vi "AttCtrlThruster.vi"(0 "ctclk":bool, 1 "Duty Cycle":dbl=1.0, 2 "Up":bool, 3 "Period":dbl=10.0, 4 "clkwis":bool, 5 "Float":bool, 6 "Angular Acceleration":u16(ring) items=["Fast", "Slow"], 7 "Left":bool, 8 "Right":bool, 9 "task in":refnum<k21>, 11 "error in":errorcluster, 13 "Down":bool) -> (10 "task out":refnum<k21>, 15 "error out":errorcluster)   [LabVIEW 2012]
panel:
  # "Attitude Control"
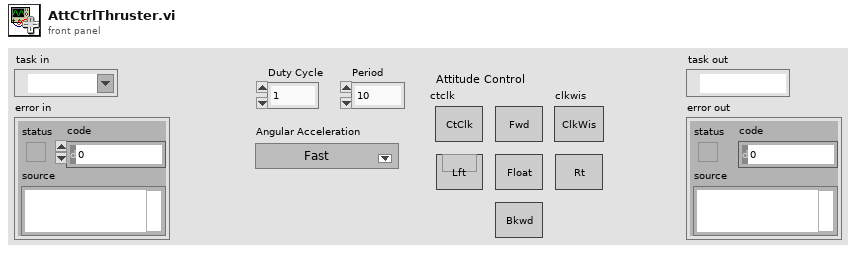
[diagram p1: front panel]
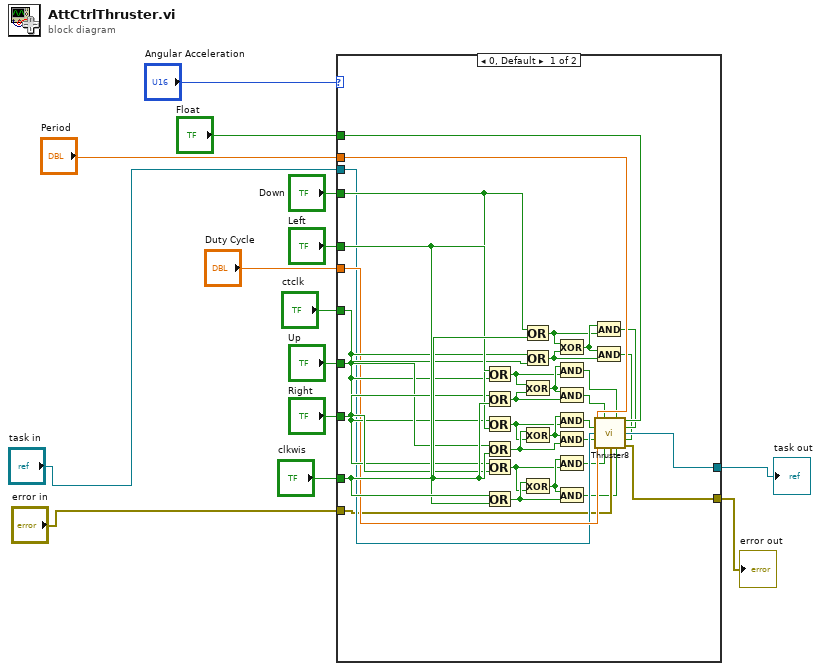
[diagram p0: block diagram]
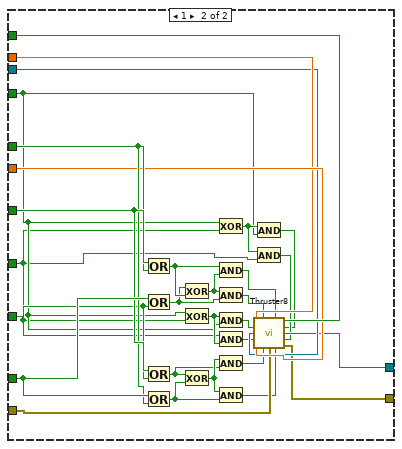
[diagram p2: hidden frame]
diagram:
  n1 = case shown="0, Default" "Angular Acceleration" {
    tunnel: "Float" -> [w47 w76]
    tunnel: "Down" -> [w44 w56]
    tunnel: "Left" -> [w45 w73]
    tunnel: "Up" -> [w42 w54]
    tunnel: "Right" -> [w43 w72]
    tunnel: "clkwis" -> [w46 w75]
    tunnel: "ctclk" -> [w41 w74]
    tunnel: "Duty Cycle" -> [w40 w71]
    tunnel: "Period" -> [w39 w70]
    tunnel: "task in" -> [w38 w68]
    tunnel: "error in" -> [w37 w69]
    tunnel: [w36 w67] -> w4
    tunnel: [w35 w66] -> w3
    frame 0, Default {
      n2 = Or(x=w45, y=w41) -> (x .or. y?=w30:bool)
      n3 = Or(x=w43, y=w46) -> (x .or. y?=w28:bool)
      n4 = Or(x=w41, y=w44) -> (x .or. y?=w16:bool)
      n5 = Or(x=w42, y=w46) -> (x .or. y?=w18:bool)
      n6 = Or(x=w41, y=w43) -> (x .or. y?=w20:bool)
      n7 = Or(x=w46, y=w45) -> (x .or. y?=w22:bool)
      n8 = Or(x=w44, y=w46) -> (x .or. y?=w26:bool)
      n9 = Or(x=w41, y=w42) -> (x .or. y?=w24:bool)
      n10 = Exclusive Or(1:w28, 2:w30) -> (0:w34:bool)
      n11 = Exclusive Or(1:w16, 2:w18) -> (0:w31:bool)
      n12 = Exclusive Or(1:w20, 2:w22) -> (0:w32:bool)
      n13 = Exclusive Or(1:w24, 2:w26) -> (0:w33:bool)
      n14 = And(x=w34, y=w30) -> (x .and. y?=w29:bool)
      n15 = And(x=w34, y=w28) -> (x .and. y?=w27:bool)
      n16 = And(x=w31, y=w16) -> (x .and. y?=w15:bool)
      n17 = And(x=w31, y=w18) -> (x .and. y?=w17:bool)
      n18 = And(x=w32, y=w20) -> (x .and. y?=w19:bool)
      n19 = And(x=w32, y=w22) -> (x .and. y?=w21:bool)
      n20 = And(x=w33, y=w26) -> (x .and. y?=w25:bool)
      n21 = And(x=w33, y=w24) -> (x .and. y?=w23:bool)
      n22 = call "Thruster8.vi"("period"=w39, "Thruster 2"=w27, "Truster1"=w29, "Floating"=w47, "Thruster 3"=w15, "Thruster 8"=w25, "task in"=w38, "Thruster 4"=w17, "Thruster 7"=w23, "Duty Cycle"=w40, "Thruster 5"=w19, "error in"=w37, "Thruster 6"=w21) -> ("task out"=w36:refnum<k21>, "error out"=w35:errorcluster)  [unwired: 1 in]
    }
    frame 1 {
      n23 = Or(x=w74, y=w73) -> (x .or. y?=w51:bool)
      n24 = Or(x=w75, y=w72) -> (x .or. y?=w49:bool)
      n25 = Or(x=w74, y=w72) -> (x .or. y?=w61:bool)
      n26 = Or(x=w75, y=w73) -> (x .or. y?=w59:bool)
      n27 = Exclusive Or(1:w51, 2:w49) -> (0:w52:bool)
      n28 = Exclusive Or(1:w54, 2:w56) -> (0:w57:bool)
      n29 = Exclusive Or(1:w59, 2:w61) -> (0:w62:bool)
      n30 = Exclusive Or(1:w54, 2:w56) -> (0:w65:bool)
      n31 = And(x=w51, y=w52) -> (x .and. y?=w50:bool)
      n32 = And(x=w52, y=w49) -> (x .and. y?=w48:bool)
      n33 = And(x=w57, y=w56) -> (x .and. y?=w55:bool)
      n34 = And(x=w54, y=w57) -> (x .and. y?=w53:bool)
      n35 = And(x=w62, y=w61) -> (x .and. y?=w60:bool)
      n36 = And(x=w62, y=w59) -> (x .and. y?=w58:bool)
      n37 = And(x=w65, y=w56) -> (x .and. y?=w63:bool)
      n38 = And(x=w65, y=w54) -> (x .and. y?=w64:bool)
      n39 = call "Thruster8.vi"("period"=w70, "Thruster 2"=w48, "Truster1"=w50, "Floating"=w76, "Thruster 3"=w55, "Thruster 8"=w63, "task in"=w68, "Thruster 4"=w53, "Thruster 7"=w64, "Duty Cycle"=w71, "Thruster 5"=w60, "error in"=w69, "Thruster 6"=w58) -> ("task out"=w67:refnum<k21>, "error out"=w66:errorcluster)  [unwired: 1 in]
    }
  }
  "task out" <- w4
  "error out" <- w3
